vi "DIAdem Daemon Control.vi"(4 "error in (no error)":errorcluster, 6 "DD Startup Tmo (60000 ms)":u32=60000, 7 "Action (START)":enum16{"START", "STOP", "STATUS"}(ring)) -> (0 "error out":errorcluster, 3 "Daemon State":T1(ring))   [LabVIEW 2011]
uses:
  lib/DIAdem Daemon Queue.ctl
  lib/DIAdem Daemon Script Type.ctl
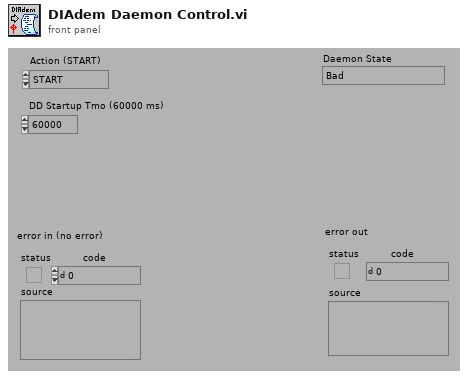
[diagram p1: front panel]
types:
  T1 = enum32{"Bad", "Idle", "Run top level", "Running"}
  T2 = typedef "DIAdem Daemon Queue.ctl" = cluster{"Report Template TDM":path, "Report Processor VBS":path, "Report Path PDF":path, "Report Script Params":string, "Username":string, "Script Type":T3, "Report Query Params":string, "Client Machine":string, "Print on Client?":bool, "Response Queue Name":string, "Script Variables":string[], "Start Request Time":timestamp, "Wait?":bool}
  T3 = typedef "DIAdem Daemon Script Type.ctl" = enum16{"Report", "Query", "Script", "Datasheet", "Append", "Restart", "Stop"}
  T4 = typedef "Rendezvous RefNum" = refnum<k1>
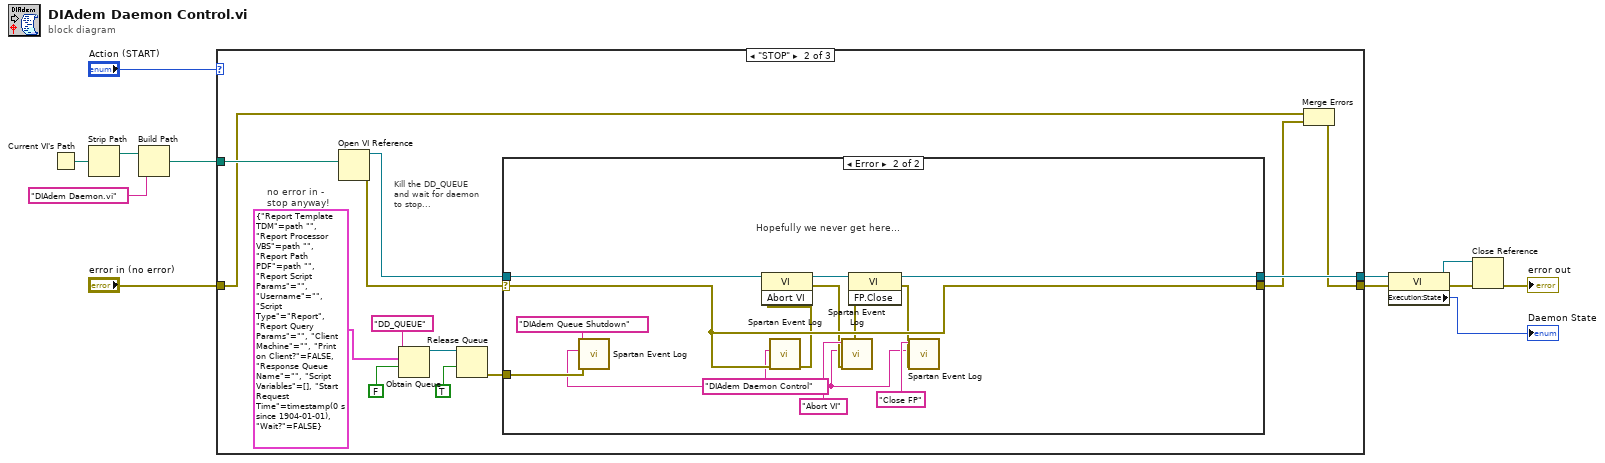
[diagram p0: block diagram]
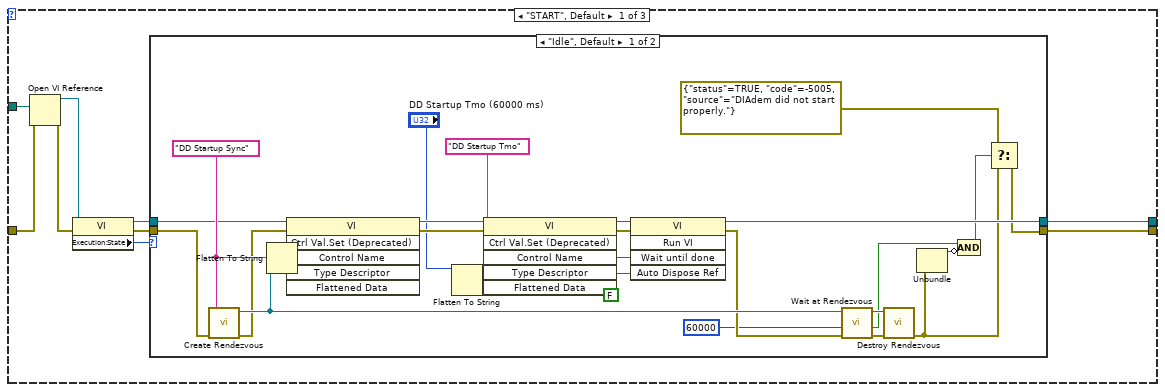
[diagram p2: hidden frame]
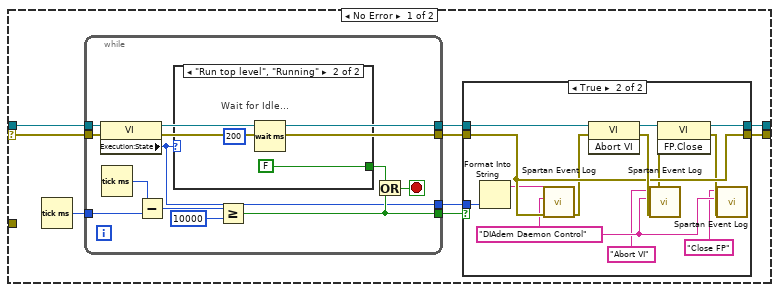
[diagram p4: hidden frame]
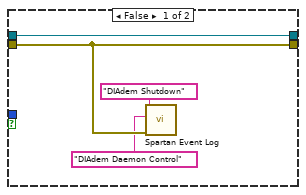
[diagram p5: hidden frame]
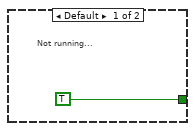
[diagram p6: hidden frame]
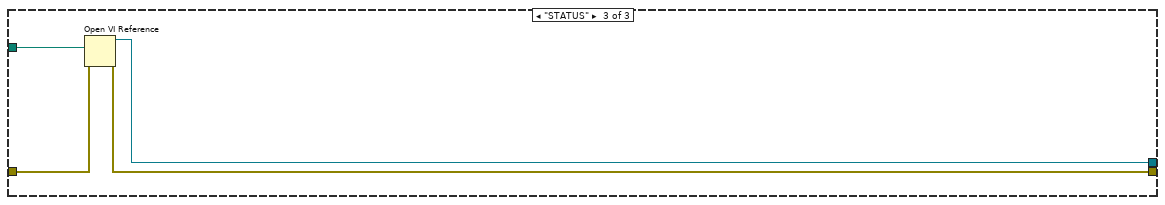
[diagram p7: hidden frame]
diagram:
  n1 = Current VI's Path() -> (path=w12:path)
  n2 = Strip Path(path=w12) -> (stripped path=w11:path)  [unwired: 1 out]
  n3 = Build Path(base path=w11, name or relative path="DIAdem Daemon.vi") -> (appended path=w2:path)
  n4 = case shown="\"STOP\"" "Action (START)" {
    tunnel: "error in (no error)" -> [w19 w53 w121]
    tunnel: [w21 w51 w120] -> w5
    tunnel: [w20 w63 w118] -> w7
    tunnel: w2 -> [w18 w62 w119]
    frame "START", Default {
      n5 = Open VI Reference(vi path=w18, error in (no error)=w19) -> (vi reference=w17:refnum<vi>, error out=w16:errorcluster)  [unwired: 4 out]
      n6 = property class="VI"(reference=w17, error in=w16) -> (reference out=w13:refnum<vi>, error out=w15:errorcluster, "Execution:State"=w14:T1)
      n7 = case shown="\"Idle\", Default" w14 {
        tunnel: [w35 w49] -> w21
        tunnel: [w38 w50] -> w20
        tunnel: w15 -> [w28 w49]
        tunnel: w13 -> [w37 w50]
        frame "Idle", Default {
          w43 = FALSE
          w48 = "DD Startup Sync"
          n8 = call <vilib>:"Create Rendezvous.vi"("error in (no error)"=w28, "name (unnamed)"=w48) -> ("error out"=w44:errorcluster, "rendezvous"=w45:T4)  [unwired: 1 in, 3 out]
          n9 = Flatten To String(anything=w45) -> (data string=w46:string, type string=w47:i16[])  [unwired: 1 in, 3 out]
          n10 = invoke class="VI" method="Ctrl Val.Set (Deprecated)"(reference=w37, error in=w44, "Control Name"=w48, "Type Descriptor"=w47, "Flattened Data"=w46) -> (reference out=w27:refnum<vi>, error out=w26:errorcluster)  [unwired: 1 in, 4 out]
          n11 = Flatten To String(anything="DD Startup Tmo (60000 ms)") -> (data string=w23:string, type string=w24:i16[])  [unwired: 1 in, 3 out]
          n12 = invoke class="VI" method="Ctrl Val.Set (Deprecated)"(reference=w27, error in=w26, "Control Name"="DD Startup Tmo", "Type Descriptor"=w24, "Flattened Data"=w23) -> (reference out=w30:refnum<vi>, error out=w29:errorcluster)  [unwired: 1 in, 4 out]
          n13 = invoke class="VI" method="Run VI"(reference=w30, error in=w29, "Wait until done"=w43, "Auto Dispose Ref"=w43) -> (reference out=w38:refnum<vi>, error out=w42:errorcluster)  [unwired: 1 in, 3 out]
          n14 = call <vilib>:"Wait at Rendezvous.vi"("error in (no error)"=w42, "ms timeout (-1)"=60000, "rendezvous"=w45) -> ("error out"=w40:errorcluster, "timed out"=w33:bool, "rendezvous out"=w39:T4)  [unwired: 2 out]
          n15 = call <vilib>:"Destroy Rendezvous.vi"("error in (no error)"=w40, "rendezvous"=w39) -> ("error out"=w36:errorcluster)  [unwired: 5 out]
          n16 = Unbundle(w36) -> ("status"=w34:bool)  [unwired: 2 out]
          n17 = Compound Arithmetic op=AND(w33, invert w34) -> (w32:bool)
          n18 = Select(t=errorcluster {"status"=TRUE, "code"=-5005, "source"="DIAdem did not start properly."}, s=w32, f=w36) -> (s? t:f=w35:errorcluster)
        }
        frame "Run top level", "Running" {
        }
      }
    }
    frame "STOP" {
      # "Kill the DD_QUEUE\nand wait for daemon\nto stop..."
      # "no error in -\nstop anyway!"
      n19 = Open VI Reference(vi path=w62) -> (vi reference=w61:refnum<vi>, error out=w60:errorcluster)  [unwired: 1 in, 4 out]
      n20 = Obtain Queue(name (unnamed)="DD_QUEUE", element data type=T2 {"Report Template TDM"=path "", "Report Processor VBS"=path "", "Report Path PDF"=path "", "Report Script Params"="", "Username"="", "Script Type"=enum."Report", "Report Query Params"="", "Client Machine"="", "Print on Client?"=FALSE, "Response Queue Name"="", "Script Variables"=[], "Start Request Time"=timestamp(0 s since 1904-01-01), "Wait?"=FALSE} ("DD_Report"), create if not found? (T)=FALSE) -> (queue out=w57:refnum<queue>)  [unwired: 2 in, 2 out]
      n21 = Release Queue(queue=w57, force destroy? (F)=TRUE) -> (error out=w59:errorcluster)  [unwired: 1 in, 2 out]
      n22 = case shown="Error" w60 {
        selector: w60 -> [w71 w114]
        tunnel: [w68 w115] -> w63
        tunnel: [w67 w114] -> w52
        tunnel: w61 -> [w72 w117]
        tunnel: w59 -> [_ w109]
        frame No Error {
          n23 = Tick Count (ms)() -> (millisecond timer value=w66:u32)
          n24 = while {
            tunnel: [w100] -> w69
            tunnel: [w99] -> w70
            tunnel: w71 -> [w101]
            tunnel: w72 -> [w98]
            tunnel: [w92] -> w65
            tunnel: w66 -> [w96]
            tunnel: [w90] -> w64
            stop <- w91 stop-if-true
            n25 = property class="VI"(reference=w98, error in=w101) -> (reference out=w100:refnum<vi>, error out=w99:errorcluster, "Execution:State"=w90:T1)
            n26 = Tick Count (ms)() -> (millisecond timer value=w97:u32)
            n27 = Subtract(x=w97, y=w96) -> (x-y=w95:u32)
            n28 = case shown="\"Run top level\", \"Running\"" w90 {
              tunnel: [TRUE FALSE] -> w93
              frame Default {
                # "Not running..."
              }
              frame "Run top level", "Running" {
                # "Wait for Idle..."
                n29 = Wait (ms)(milliseconds to wait=u32 200) -> ()  [unwired: 1 out]
              }
            }
            n30 = Greater Or Equal?(x=w95, y=u32 10000) -> (x >= y?=w92:bool)
            n31 = Or(x=w93, y=w92) -> (x .or. y?=w91:bool)
          }
          n32 = case shown="True" w65 {
            tunnel: w70 -> [w75 w85]
            tunnel: w69 -> [w76 w89]
            tunnel: [w76 w87] -> w68
            tunnel: [w75 w85] -> w67
            tunnel: w64 -> [_ w83]
            frame False {
              n33 = call "Spartan Event Log.vi"("error in (no error)"=w75, "module (\"\")"="DIAdem Daemon Control" ("module (\"\")"), "message (\"\")"="DIAdem Shutdown" ("message (\"\")")) -> ()  [unwired: 2 in, 4 out]
            }
            frame True {
              w81 = "DIAdem Daemon Control" ("module (\"\")")
              n34 = Format Into String(w83) -> (resulting string=w82:string)  [unwired: 3 in, 1 out]
              n35 = call "Spartan Event Log.vi"("error in (no error)"=w85, "module (\"\")"=w81, "message (\"\")"=w82) -> ("error out"=w78:errorcluster)  [unwired: 2 in, 3 out]
              n36 = invoke class="VI" method="Abort VI"(reference=w89, error in=w78) -> (reference out=w88:refnum<vi>, error out=w86:errorcluster)  [unwired: 1 in, 1 out]
              n37 = call "Spartan Event Log.vi"("error in (no error)"=w86, "module (\"\")"=w81, "message (\"\")"="Abort VI" ("message (\"\")")) -> ("error out"=w77:errorcluster)  [unwired: 2 in, 3 out]
              n38 = invoke class="VI" method="FP.Close"(reference=w88, error in=w77) -> (reference out=w87:refnum<vi>, error out=w84:errorcluster)  [unwired: 1 in, 1 out]
              n39 = call "Spartan Event Log.vi"("error in (no error)"=w84, "module (\"\")"=w81, "message (\"\")"="Close FP" ("message (\"\")")) -> ()  [unwired: 2 in, 4 out]
            }
          }
        }
        frame Error {
          w108 = "DIAdem Daemon Control" ("module (\"\")")
          # "Hopefully we never get here..."
          n40 = call "Spartan Event Log.vi"("error in (no error)"=w109, "module (\"\")"=w108, "message (\"\")"="DIAdem Queue Shutdown" ("message (\"\")")) -> ()  [unwired: 2 in, 4 out]
          n41 = call "Spartan Event Log.vi"("error in (no error)"=w114, "module (\"\")"=w108) -> ("error out"=w106:errorcluster)  [unwired: 3 in, 3 out]
          n42 = invoke class="VI" method="Abort VI"(reference=w117, error in=w106) -> (reference out=w116:refnum<vi>, error out=w110:errorcluster)  [unwired: 1 in, 1 out]
          n43 = call "Spartan Event Log.vi"("error in (no error)"=w110, "module (\"\")"=w108, "message (\"\")"="Abort VI" ("message (\"\")")) -> ("error out"=w105:errorcluster)  [unwired: 2 in, 3 out]
          n44 = invoke class="VI" method="FP.Close"(reference=w116, error in=w105) -> (reference out=w115:refnum<vi>, error out=w111:errorcluster)  [unwired: 1 in, 1 out]
          n45 = call "Spartan Event Log.vi"("error in (no error)"=w111, "module (\"\")"=w108, "message (\"\")"="Close FP" ("message (\"\")")) -> ()  [unwired: 2 in, 4 out]
        }
      }
      n46 = Merge Errors(w53, w52) -> (w51:errorcluster)
    }
    frame "STATUS" {
      n47 = Open VI Reference(vi path=w119, error in (no error)=w121) -> (vi reference=w118:refnum<vi>, error out=w120:errorcluster)  [unwired: 4 out]
    }
  }
  n48 = property class="VI"(reference=w7, error in=w5) -> (reference out=w8:refnum<vi>, error out=w4:errorcluster, "Execution:State"=→"Daemon State":T1)
  n49 = Close Reference(reference=w8, error in (no error)=w4) -> (error out=→"error out":errorcluster)
